vi "Cleanup.vi"(8 "error in (no error)":errorcluster, 11 "WriteCommand in":refnum<class "WriteCommand.lvclass">) -> (0 "error out":errorcluster, 3 "WriteCommand out":refnum<class "WriteCommand.lvclass">)   [LabVIEW 2023, in "HAF.lvlib" / "WriteCommand.lvclass"]
doc: "Ensures a clean and controlled stop of the Command's Driver."
uses:
  WriteCommand.lvclass
  WriteCommand.lvclass/WriteCommand.ctl
  Driver/Driver.lvclass
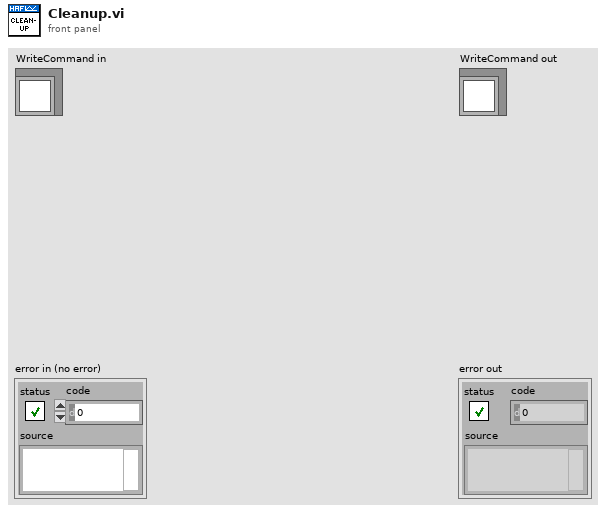
[diagram p1: front panel]
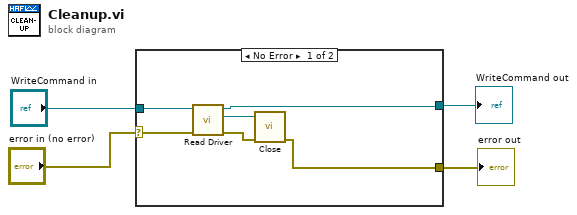
[diagram p0: block diagram]
diagram:
  n1 = case shown="No Error" "error in (no error)" {
    selector: "error in (no error)" -> [w9 w12]
    tunnel: [w5 w12] -> w3
    tunnel: [w6 w11] -> w1
    tunnel: "WriteCommand in" -> [w10 w11]
    frame No Error {
      n2 = call-dynamic "Read Driver.vi"("error in (no error)"=w9, "WriteCommand in"=w10) -> ("error out"=w7:errorcluster, "Driver"=w8:refnum<class "Driver.lvclass">, "WriteCommand out"=w6:refnum<class "WriteCommand.lvclass">)  [unwired: 7 in]
      n3 = call-dynamic "Close.vi"("error in (no error)"=w7, "Driver in"=w8) -> ("error out"=w5:errorcluster)  [unwired: 8 in, 1 out]
    }
    frame Error {
    }
  }
  "error out" <- w3
  "WriteCommand out" <- w1
